vi "Test Build SeqEdit Execution Plan.vi"() -> (0 "error out":errorcluster)   [LabVIEW 2025]
doc: "This VI tests the logic for building execution plans to launch TestStand Sequence Editor with and without environment arguments."
uses:
  src/TSDiscovery Mock/TSDiscovery Mock.lvclass
  <vilib>/addons/_JKI Toolkits/Caraya/classes/Test/Test.lvclass
  <vilib>/addons/_JKI Toolkits/Caraya/classes/Assert/Assert.lvclass
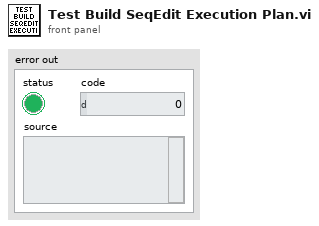
[diagram p1: front panel]
types:
  T1 = enum16{"open", "replace", "create", "open or create", "replace or create", "replace or create with confirmation"}
  T2 = typedef "TSInstall--cluster.ctl" = cluster{"Version":string, "Architecture":T3, "Version Key":string, "ID":string}
  T3 = typedef "Architecture--enum.ctl" = enum16{"32bit", "64bit"}
  T4 = typedef "Execution Plan--cluster.ctl" = cluster{"Exe Path":path, "Args":string[], "Timeout":i32}
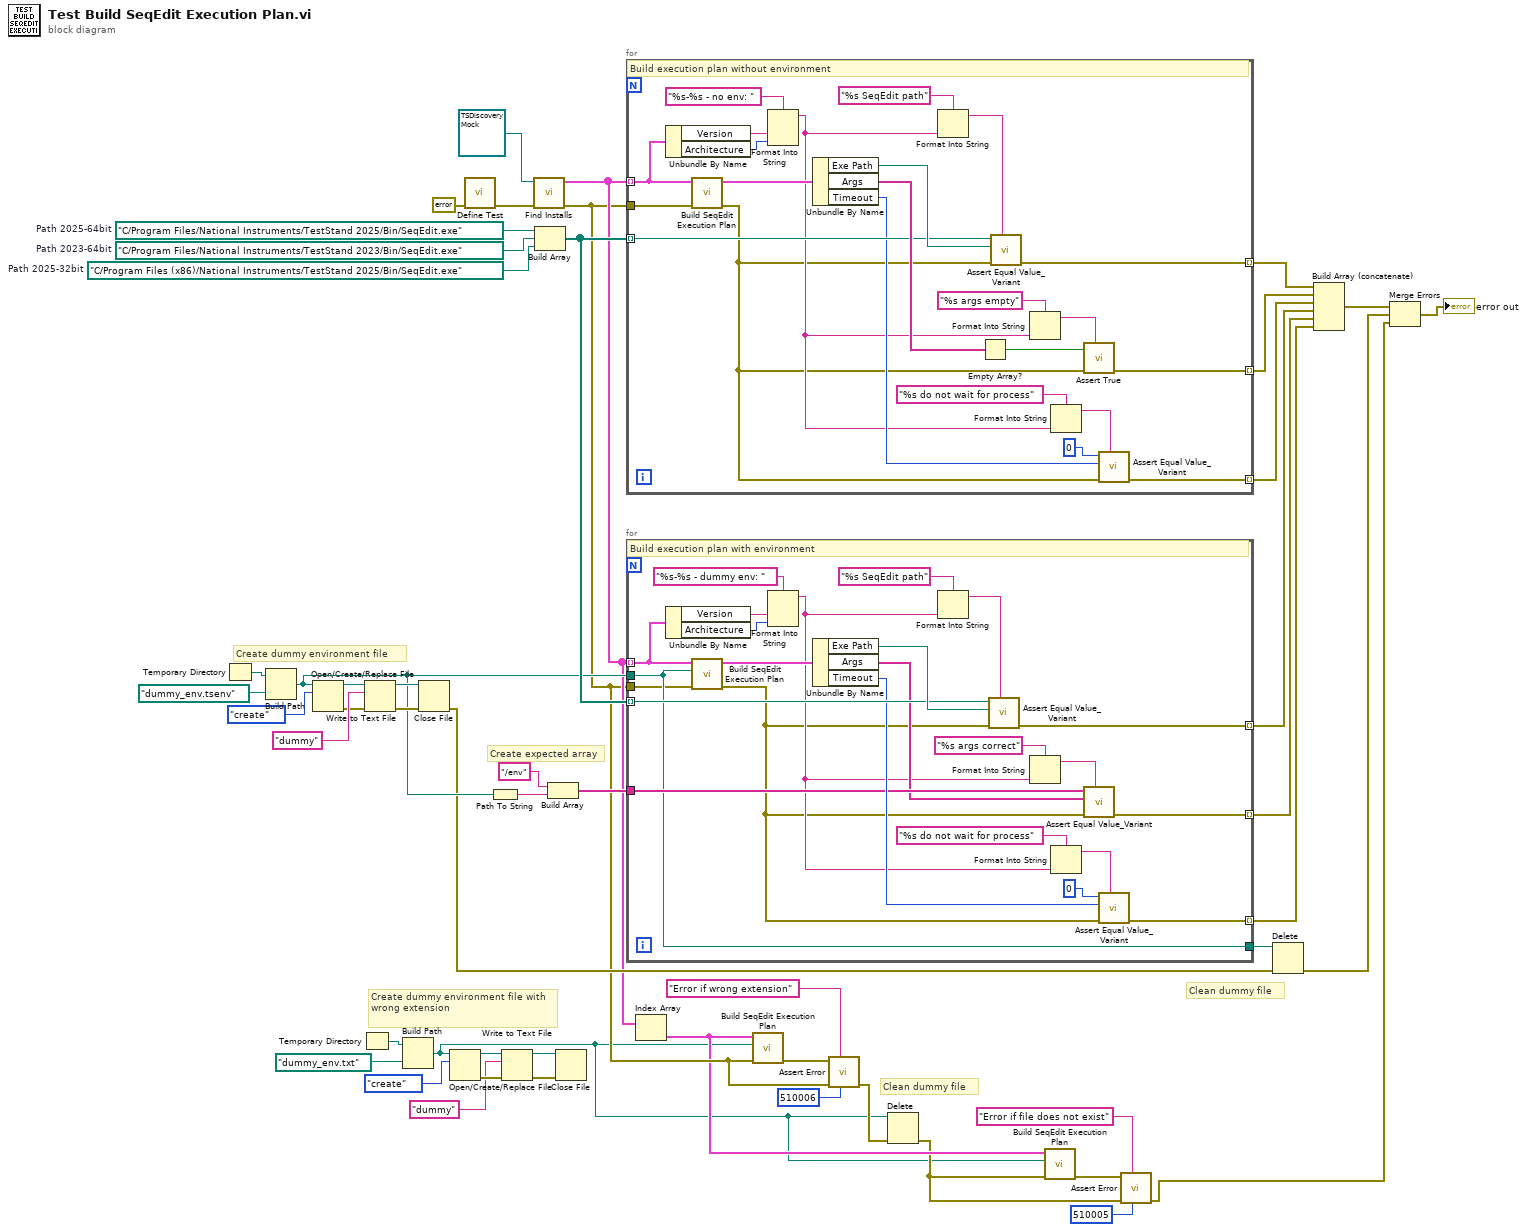
[diagram p0: block diagram]
diagram:
  w46 = path "C:/Program Files (x86)/National Instruments/TestStand 2025/Bin/SeqEdit.exe"  # Path 2025-32bit
  w47 = path "C:/Program Files/National Instruments/TestStand 2023/Bin/SeqEdit.exe"  # Path 2023-64bit
  w48 = path "C:/Program Files/National Instruments/TestStand 2025/Bin/SeqEdit.exe"  # Path 2025-64bit
  # "Clean dummy file"
  # "Create dummy environment file with wrong extension"
  # "Clean dummy file"
  # "Create expected array"
  # "Create dummy environment file"
  n1 = Temporary Directory() -> (w37:path)
  n2 = Build Path(base path=w37, name or relative path=path "dummy_env.tsenv") -> (appended path=w26:path)
  n3 = Open/Create/Replace File(file path (use dialog)=w26, operation (0:open)=T1."create") -> (refnum out=w33:refnum<file>, error out=w28:errorcluster)  [unwired: 4 in, 1 out]
  n4 = Temporary Directory() -> (w21:path)
  n5 = Write to Text File(file (use dialog)=w33, text="dummy", error in=w28) -> (refnum out=w32:refnum<file>, error out=w27:errorcluster)  [unwired: 1 in, 1 out]
  n6 = Build Path(base path=w21, name or relative path=path "dummy_env.txt") -> (appended path=w1:path)
  n7 = Close File(refnum=w32, error in=w27) -> (error out=w22:errorcluster)  [unwired: 1 out]
  n8 = Open/Create/Replace File(file path (use dialog)=w1, operation (0:open)=T1."create") -> (refnum out=w18:refnum<file>, error out=w16:errorcluster)  [unwired: 4 in, 1 out]
  n9 = call <vilib>:"Define Test.vi"("error in (no error)"=errorcluster {"status"=FALSE, "code"=0, "source"=""}) -> ("error out"=w50:errorcluster)  [unwired: 9 in, 1 out]
  n10 = Path To String(path=w26) -> (string=w31:string)
  n11 = Write to Text File(file (use dialog)=w18, text="dummy", error in=w16) -> (refnum out=w17:refnum<file>, error out=w15:errorcluster)  [unwired: 1 in, 1 out]
  n12 = call-dynamic "Find Installs.vi"("error in"=w50, "TSDiscovery Mock in"=refnum<class "TSDiscovery Mock.lvclass"> refnum) -> ("error out"=w11:errorcluster, "TSInstalls Out"=w13:T2[])  [unwired: 8 in]
  n13 = Build Array(w48, w47, w46) -> (w42:path[])
  n14 = Build Array("/env" ("element"), w31) -> (w29:string[])
  n15 = Close File(refnum=w17, error in=w15) -> ()  [unwired: 2 out]
  n16 = for {
    tunnel: w13 -> [w74] mode=indexing
    tunnel: w42 -> [w61] mode=indexing
    tunnel: [w58] -> w45 mode=indexing
    tunnel: [w57] -> w44 mode=indexing
    tunnel: [w56] -> w43 mode=indexing
    tunnel: w11 -> [w53]
    # "Build execution plan without environment"
    n17 = Unbundle By Name(w74) -> ("Version"=w72:string, "Architecture"=w71:T3)
    n18 = call "Build SeqEdit Execution Plan.vi"("error in"=w53, "TSInstall"=w74) -> ("error out"=w52:errorcluster, "Execution Plan"=w70:T4)  [unwired: 8 in]
    n19 = Format Into String(format string="%s-%s - no env: ", w72, w71) -> (resulting string=w55:string)  [unwired: 2 in, 1 out]
    n20 = Unbundle By Name(w70) -> ("Exe Path"=w62:path, "Args"=w65:string[], "Timeout"=w60:i32)
    n21 = Format Into String(format string="%s SeqEdit path", w55) -> (resulting string=w68:string)  [unwired: 2 in, 1 out]
    n22 = Empty Array?(array=w65) -> (empty?=w64:bool)
    n23 = call <vilib>:"Assert Equal Value_Variant.vi"("Label"=w68, "error in (no error)"=w52, "Actual"=w62, "Expected"=w61) -> ("error out"=w58:errorcluster)  [unwired: 6 in, 1 out]
    n24 = Format Into String(format string="%s args empty", w55) -> (resulting string=w66:string)  [unwired: 2 in, 1 out]
    n25 = Format Into String(format string="%s do not wait for process", w55) -> (resulting string=w54:string)  [unwired: 2 in, 1 out]
    n26 = call <vilib>:"Assert True.vi"("Label"=w66, "error in (no error)"=w52, "True?"=w64) -> ("error out"=w57:errorcluster)  [unwired: 7 in, 1 out]
    n27 = call <vilib>:"Assert Equal Value_Variant.vi"("Label"=w54, "error in (no error)"=w52, "Actual"=w60, "Expected"=0) -> ("error out"=w56:errorcluster)  [unwired: 6 in, 1 out]
  }
  n28 = for {
    tunnel: w13 -> [w98] mode=indexing
    tunnel: w42 -> [w87] mode=indexing
    tunnel: [w84] -> w39 mode=indexing
    tunnel: [w83] -> w40 mode=indexing
    tunnel: [w82] -> w41 mode=indexing
    tunnel: w26 -> [w77]
    tunnel: w29 -> [w81]
    tunnel: w11 -> [w76]
    tunnel: [w77] -> w24
    # "Build execution plan with environment"
    n29 = Unbundle By Name(w98) -> ("Version"=w96:string, "Architecture"=w95:T3)
    n30 = call "Build SeqEdit Execution Plan.vi"("error in"=w76, "Environment"=w77, "TSInstall"=w98) -> ("error out"=w75:errorcluster, "Execution Plan"=w94:T4)  [unwired: 7 in]
    n31 = Format Into String(format string="%s-%s - dummy env: ", w96, w95) -> (resulting string=w79:string)  [unwired: 2 in, 1 out]
    n32 = Unbundle By Name(w94) -> ("Exe Path"=w88:path, "Args"=w80:string[], "Timeout"=w86:i32)
    n33 = Format Into String(format string="%s SeqEdit path", w79) -> (resulting string=w92:string)  [unwired: 2 in, 1 out]
    n34 = call <vilib>:"Assert Equal Value_Variant.vi"("Label"=w92, "error in (no error)"=w75, "Actual"=w88, "Expected"=w87) -> ("error out"=w84:errorcluster)  [unwired: 6 in, 1 out]
    n35 = Format Into String(format string="%s args correct", w79) -> (resulting string=w90:string)  [unwired: 2 in, 1 out]
    n36 = Format Into String(format string="%s do not wait for process", w79) -> (resulting string=w78:string)  [unwired: 2 in, 1 out]
    n37 = call <vilib>:"Assert Equal Value_Variant.vi"("Label"=w90, "error in (no error)"=w75, "Actual"=w80, "Expected"=w81) -> ("error out"=w83:errorcluster)  [unwired: 6 in, 1 out]
    n38 = call <vilib>:"Assert Equal Value_Variant.vi"("Label"=w78, "error in (no error)"=w75, "Actual"=w86, "Expected"=0) -> ("error out"=w82:errorcluster)  [unwired: 6 in, 1 out]
  }
  n39 = Index Array(array=w13) -> (element=w4:T2)  [unwired: 1 in]
  n40 = call "Build SeqEdit Execution Plan.vi"("error in"=w11, "Environment"=w1, "TSInstall"=w4) -> ("error out"=w12:errorcluster)  [unwired: 7 in, 1 out]
  n41 = call <vilib>:"Assert Error.vi"("error code (1)"=510006, "Label"="Error if wrong extension", "error in (no error)"=w11, "Error?"=w12) -> ("error out"=w8:errorcluster)  [unwired: 6 in, 1 out]
  n42 = Delete(path (use dialog)=w1, error in=w8) -> (error out=w3:errorcluster)  [unwired: 3 in, 2 out]
  n43 = call "Build SeqEdit Execution Plan.vi"("error in"=w3, "Environment"=w1, "TSInstall"=w4) -> ("error out"=w7:errorcluster)  [unwired: 7 in, 1 out]
  n44 = call <vilib>:"Assert Error.vi"("error code (1)"=510005, "Label"="Error if file does not exist", "error in (no error)"=w3, "Error?"=w7) -> ("error out"=w2:errorcluster)  [unwired: 6 in, 1 out]
  n45 = Delete(path (use dialog)=w24, error in=w22) -> (error out=w23:errorcluster)  [unwired: 3 in, 2 out]
  n46 = Build Array (concatenate)(w45, w44, w43, w39, w40, w41) -> (w38:errorcluster[])
  n47 = Merge Errors(w38, w23, w2) -> (→"error out":errorcluster)
